vi "Set_Dir.vi"(8 "error in (no error)":errorcluster, 10 "Direction":bool, 11 "Lifter_motor in":refnum<class "Lifter_motor.lvclass">) -> (0 "error out":errorcluster, 2 "Driver ACK?":bool, 3 "Lifter_motor out":refnum<class "Lifter_motor.lvclass">)   [LabVIEW 2019, in "Lifter_motor.lvclass"]
uses:
  Lifter_motor.lvclass
  Lifter_motor.lvclass/Lifter_motor.ctl
  TCP Class/LifterTCP.lvclass
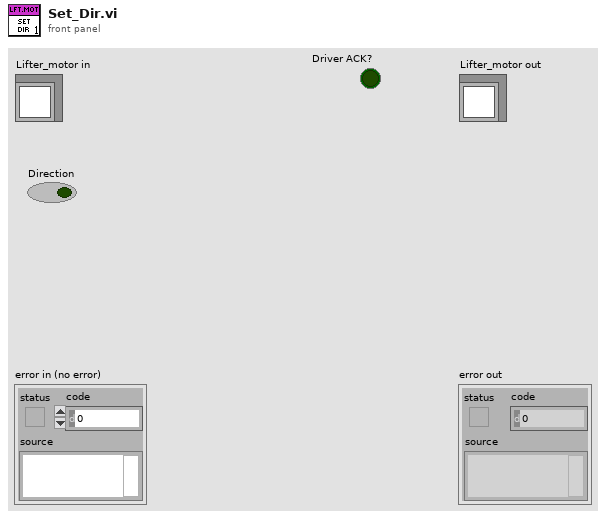
[diagram p1: front panel]
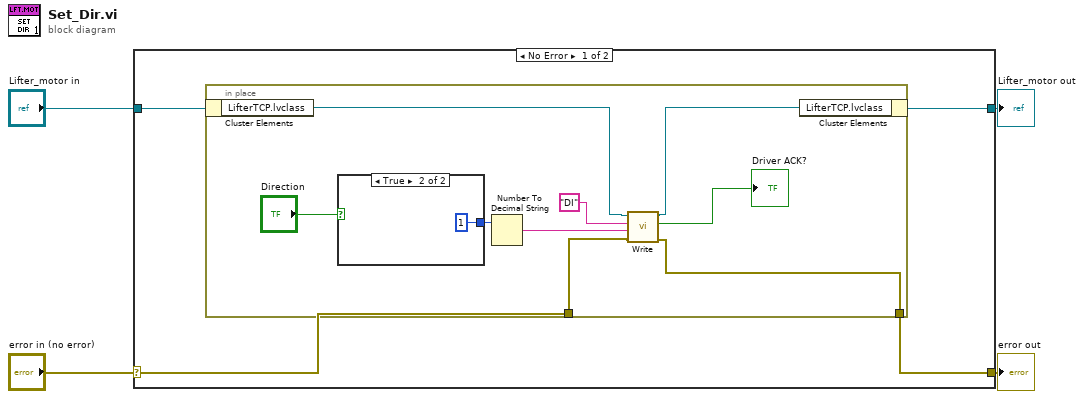
[diagram p0: block diagram]
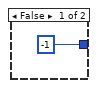
[diagram p2: hidden frame]
diagram:
  n1 = case shown="No Error" "error in (no error)" {
    selector: "error in (no error)" -> [w6 w21]
    tunnel: [w5 w21] -> w3
    tunnel: [w7 w20] -> w1
    tunnel: "Lifter_motor in" -> [w8 w20]
    frame No Error {
      n2 = in-place {
        in-place-border: w6 -> [w13]
        in-place-border: [w12] -> w5
        n3 = in-place-cluster #1(w8) -> ("LifterTCP.lvclass"=w15:refnum<class "LifterTCP.lvclass">)
        n4 = case shown="True" "Direction" {
          tunnel: [-1 ("number") 1 ("number")] -> w17
          frame False {
          }
          frame True {
          }
        }
        n5 = Number To Decimal String(number=w17) -> (decimal integer string=w9:string)  [unwired: 1 in]
        n6 = call "Write.vi"("error in (no error)"=w13, "Parameter 2"=w9, "Parameter 1"="DI" ("string"), "LifterTCP in"=w15) -> ("error out"=w12:errorcluster, "Driver ACK?"=→"Driver ACK?":bool, "LifterTCP out"=w14:refnum<class "LifterTCP.lvclass">)  [unwired: 5 in]
        n7 = in-place-cluster #1("LifterTCP.lvclass"=w14) -> (w7:refnum<class "Lifter_motor.lvclass">)
      }
    }
    frame Error {
    }
  }
  "error out" <- w3
  "Lifter_motor out" <- w1
